vi "Stream From Register.vi"(8 "Error In":errorcluster, 9 "Num Bytes":u32, 10 "Address":u8, 11 "Adept Config":T1) -> (0 "Error Out":errorcluster, 2 "Data":u8[](array[numeric]), 3 "Adept Config":T1)   [LabVIEW 2011, in "LVH-Adept.lvlib"]
doc: "Stream an array of bytes from the specified register on a Digilent FPGA board."
uses:
  <vilib>/LabVIEW Hacker/Adept/LVH-Adept.lvlib
  Private/Type Defs/Device Config.ctl
  Private/Type Defs/Status.ctl
  Private/DEPP/DEPP.lvlib
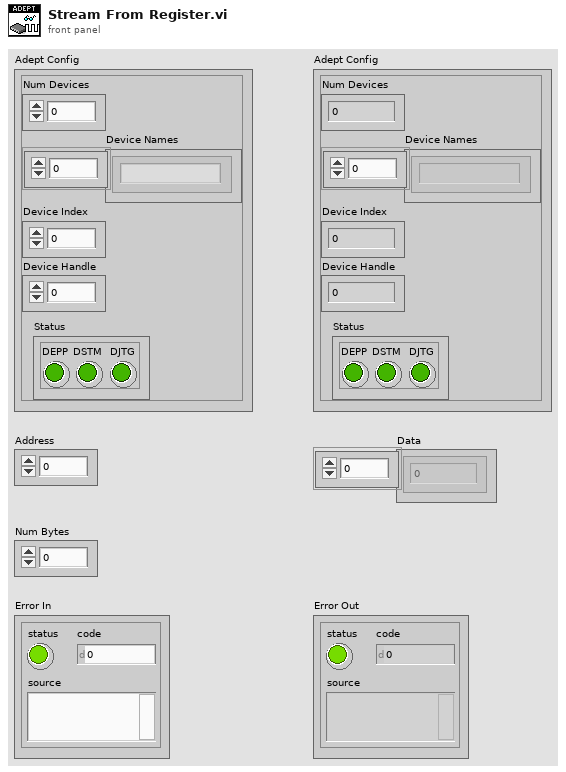
[diagram p1: front panel]
types:
  T1 = typedef "LVH-Adept.lvlib/Device Config.ctl" = cluster{"Num Devices":i32, "Device Names":string[], "Device Index":u16, "Device Handle":u32, "Status":T2}
  T2 = typedef "LVH-Adept.lvlib/Status.ctl" = cluster{"DEPP":bool, "DSTM":bool, "DJTG":bool}
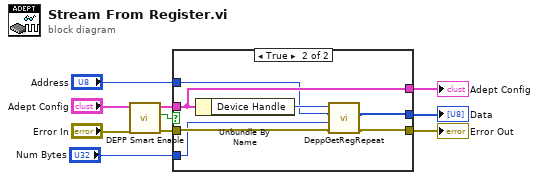
[diagram p0: block diagram]
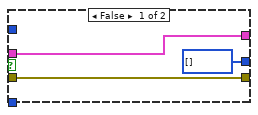
[diagram p2: hidden frame]
diagram:
  n1 = call "DEPP Smart Enable.vi"("Error In"="Error In", "Adept Config"="Adept Config") -> ("Error Out"=w8:errorcluster, "Success?"=w7:bool, "Adept Config"=w5:T1)  [unwired: 7 in]
  n2 = case shown="True" w7 {
    tunnel: w8 -> [w13 w18]
    tunnel: w5 -> [w12 w20]
    tunnel: [w13 w19] -> w6
    tunnel: [u8[] [] ("Data") w17] -> w3
    tunnel: [w12 w20] -> w4
    tunnel: "Address" -> [_ w15]
    tunnel: "Num Bytes" -> [_ w14]
    frame False {
    }
    frame True {
      n3 = Unbundle By Name(w20) -> ("Device Handle"=w16:u32)
      n4 = call "DeppGetRegRepeat.vi"("Error In"=w18, "Num Bytes"=w14, "Address"=w15, "Device Handle"=w16) -> ("Error Out"=w19:errorcluster, "Data"=w17:u8[])  [unwired: 5 in, 1 out]
    }
  }
  "Error Out" <- w6
  "Adept Config" <- w4
  "Data" <- w3
